vi "SPVM Reader.vi"(8 "error in":errorcluster, 11 "file (use dialog)":path) -> (0 "error out":errorcluster, 1 "VoxelData":u8[](array[numeric]), 3 "Metadata":T1, 4 "Length ( Bytes )":i32, 6 "cancelled":bool)   [LabVIEW 2020]
uses:
  <vilib>/Utility/error.llb/Error Cluster From Error Code.vi
  <vilib>/ErrorRing/Error Ring.xnode
panel:
  out "Scale\nunits":string
  out "Scale\nnumeric":ext
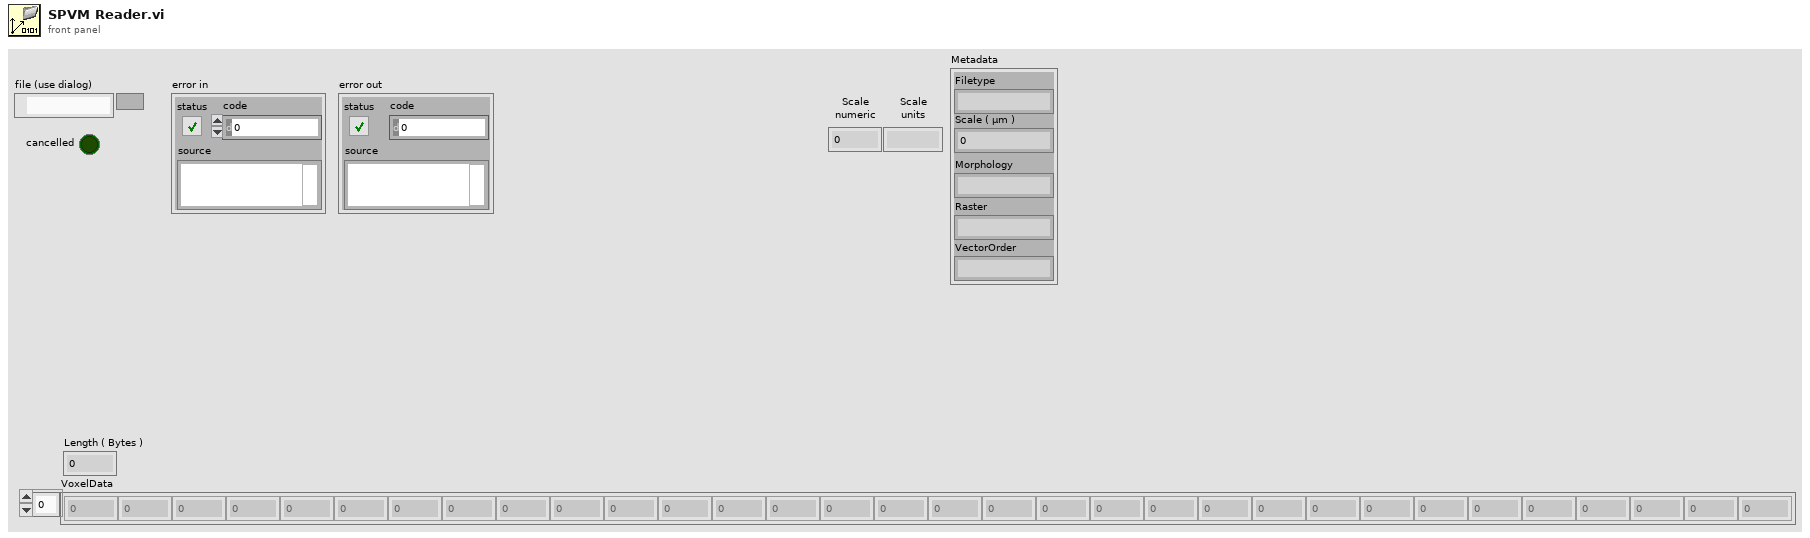
[diagram p1: front panel]
types:
  T1 = cluster{"Filetype":string, "Scale ( µm )":ext, "Morphology":string, "Raster":string, "VectorOrder":string}
  T2 = cluster{"FileType":string, "Scale ( um )":ext, "Morphology":string, "Raster":string, "VectorOrder":string}
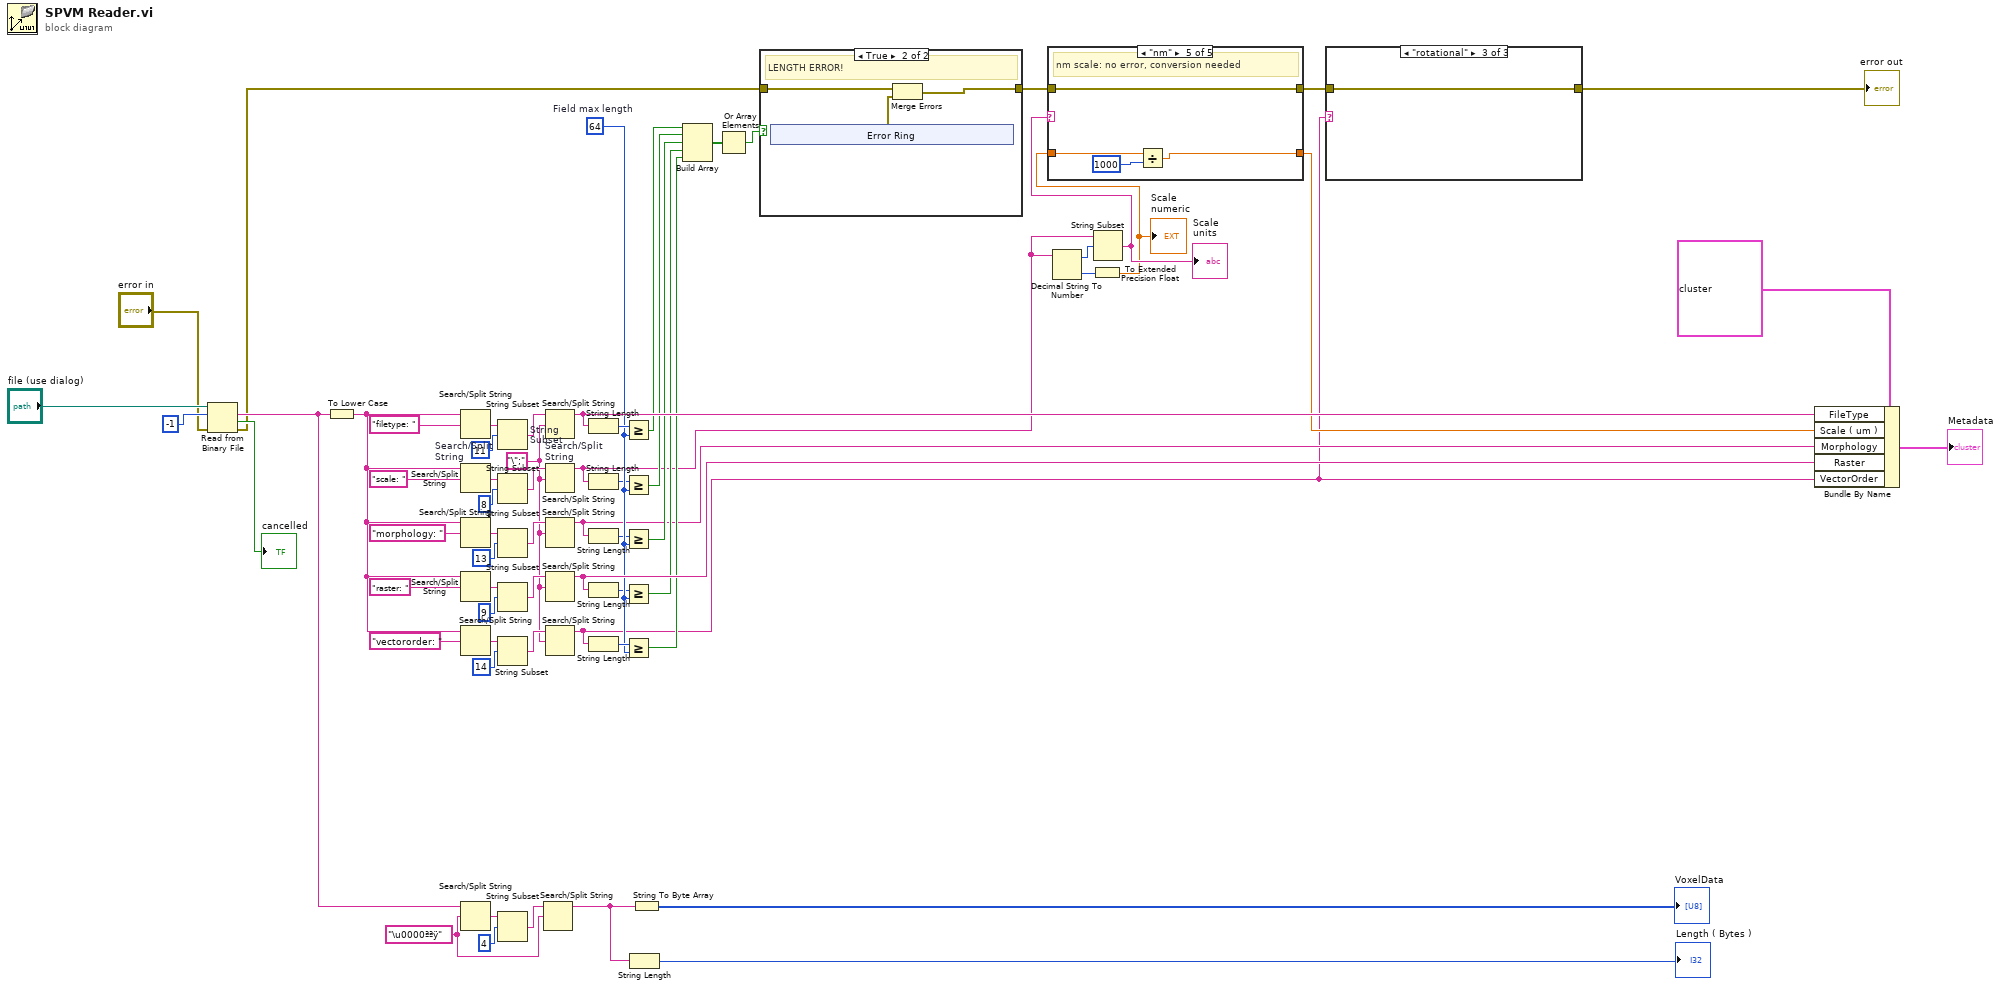
[diagram p0: block diagram]
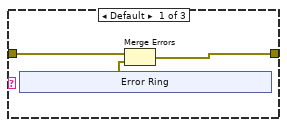
[diagram p2: hidden frame]
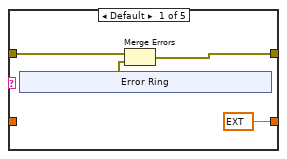
[diagram p4: hidden frame]
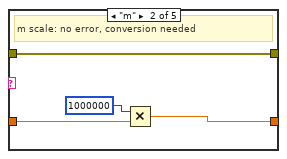
[diagram p5: hidden frame]
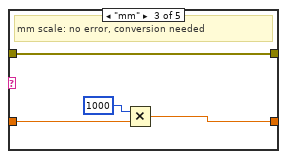
[diagram p6: hidden frame]
diagram:
  w23 = 64  # Field max length
  w29 = "\";" ("search string/char (-)")
  w63 = "\u0000ªªÿ" ("search string/char (-)")
  n1 = Read from Binary File(8:"error in", 10:-1 ("count (1)"), 11:"file (use dialog)") -> (0:w13:errorcluster, 1:→"cancelled":bool, 2:w51:string)  [unwired: 3 in, 1 out]
  n2 = To Lower Case(string=w51) -> (all lower case string=w28:string)
  n3 = Search/Split String "Search/Split\nString"(string=w28, search string/char (-)="filetype: ") -> (match + rest of string=w49:string)  [unwired: 1 in, 2 out]
  n4 = Search/Split String(string=w28, search string/char (-)="scale: ") -> (match + rest of string=w48:string)  [unwired: 1 in, 2 out]
  n5 = Search/Split String(string=w28, search string/char (-)="morphology: ") -> (match + rest of string=w47:string)  [unwired: 1 in, 2 out]
  n6 = Search/Split String(string=w28, search string/char (-)="raster: ") -> (match + rest of string=w46:string)  [unwired: 1 in, 2 out]
  n7 = Search/Split String(string=w28, search string/char (-)="vectororder: ") -> (match + rest of string=w32:string)  [unwired: 1 in, 2 out]
  n8 = Search/Split String(string=w51, search string/char (-)=w63) -> (match + rest of string=w58:string)  [unwired: 1 in, 2 out]
  n9 = String Subset "String\nSubset"(string=w49, offset (0)=11) -> (substring=w38:string)  [unwired: 1 in]
  n10 = String Subset(string=w48, offset (0)=8) -> (substring=w39:string)  [unwired: 1 in]
  n11 = String Subset(string=w47, offset (0)=13) -> (substring=w40:string)  [unwired: 1 in]
  n12 = String Subset(string=w46, offset (0)=9) -> (substring=w41:string)  [unwired: 1 in]
  n13 = String Subset(string=w32, offset (0)=14) -> (substring=w30:string)  [unwired: 1 in]
  n14 = String Subset(string=w58, offset (0)=4) -> (substring=w62:string)  [unwired: 1 in]
  n15 = Search/Split String(string=w62, search string/char (-)=w63) -> (substring before match=w35:string)  [unwired: 1 in, 2 out]
  n16 = Search/Split String "Search/Split\nString"(string=w38, search string/char (-)=w29) -> (substring before match=w27:string)  [unwired: 1 in, 2 out]
  n17 = Search/Split String(string=w39, search string/char (-)=w29) -> (substring before match=w8:string)  [unwired: 1 in, 2 out]
  n18 = Search/Split String(string=w40, search string/char (-)=w29) -> (substring before match=w2:string)  [unwired: 1 in, 2 out]
  n19 = Search/Split String(string=w41, search string/char (-)=w29) -> (substring before match=w26:string)  [unwired: 1 in, 2 out]
  n20 = Search/Split String(string=w30, search string/char (-)=w29) -> (substring before match=w1:string)  [unwired: 1 in, 2 out]
  n21 = String Length(string=w27) -> (length=w25:i32)
  n22 = String Length(string=w8) -> (length=w22:i32)
  n23 = String Length(string=w2) -> (length=w21:i32)
  n24 = String Length(string=w26) -> (length=w20:i32)
  n25 = String Length(string=w1) -> (length=w24:i32)
  n26 = Greater Or Equal?(x=w25, y=w23) -> (x >= y?=w19:bool)
  n27 = Greater Or Equal?(x=w22, y=w23) -> (x >= y?=w18:bool)
  n28 = Greater Or Equal?(x=w21, y=w23) -> (x >= y?=w17:bool)
  n29 = Greater Or Equal?(x=w20, y=w23) -> (x >= y?=w16:bool)
  n30 = Greater Or Equal?(x=w24, y=w23) -> (x >= y?=w15:bool)
  n31 = String Length(string=w35) -> (length=→"Length ( Bytes )":i32)
  n32 = String To Byte Array(string=w35) -> (unsigned byte array=→"VoxelData":u8[])
  n33 = Build Array(w19, w18, w17, w16, w15) -> (w14:bool[])
  n34 = Or Array Elements(Boolean array=w14) -> (logical OR=w12:bool)
  n35 = case shown="True" w12 {
    tunnel: w13 -> [w64 w66]
    tunnel: [w64 w67] -> w10
    frame False {
      # "No length error"
    }
    frame True {
      # "LENGTH ERROR!"
      n36 = xnode "Error Ring"() -> ("error out"=w65:errorcluster)
      n37 = Merge Errors(w66, w65) -> (w67:errorcluster)
    }
  }
  n38 = Decimal String To Number(string=w8) -> (offset past number=w11:i32, number=w9:i32)  [unwired: 2 in]
  n39 = String Subset(string=w8, offset (0)=w11) -> (substring=w6:string)  [unwired: 1 in]
  "Scale\nunits" <- w6
  n40 = To Extended Precision Float(1:w9) -> (0:w5:ext)
  "Scale\nnumeric" <- w5
  n41 = case shown="\"nm\"" w6 {
    tunnel: [ext nan w85 w89 w91 w92] -> w7
    tunnel: w5 -> [_ w84 w88 w91 w94]
    tunnel: w10 -> [w75 w82 w86 w90 w95]
    tunnel: [w76 w82 w86 w90 w95] -> w4
    frame Default {
      n42 = xnode "Error Ring"() -> ("error out"=w74:errorcluster)
      n43 = Merge Errors(w75, w74) -> (w76:errorcluster)
    }
    frame "m" {
      # "m scale: no error, conversion needed"
      n44 = Multiply(x=1000000, y=w84) -> (x*y=w85:ext)
    }
    frame "mm" {
      # "mm scale: no error, conversion needed"
      n45 = Multiply(x=1000, y=w88) -> (x*y=w89:ext)
    }
    frame "µm" {
      # "µm scale: no error, no conversion needed"
    }
    frame "nm" {
      # "nm scale: no error, conversion needed"
      n46 = Divide(x=w94, y=1000 ("x")) -> (x/y=w92:ext)
    }
  }
  n47 = case shown="\"rotational\"" w1 {
    tunnel: w4 -> [w97 w104 w105]
    tunnel: [w98 w104 w105] -> w3
    frame Default {
      n48 = xnode "Error Ring"() -> ("error out"=w96:errorcluster)
      n49 = Merge Errors(w97, w96) -> (w98:errorcluster)
    }
    frame "planar" {
    }
    frame "rotational" {
    }
  }
  "error out" <- w3
  n50 = Bundle By Name "Bundle By Name"(cluster=T2 {"FileType"="", "Scale ( um )"=0.0, "Morphology"="", "Raster"="", "VectorOrder"=""} ("input cluster"), "FileType"=w27, "Scale ( um )"=w7, "Morphology"=w2, "Raster"=w26, "VectorOrder"=w1) -> (→"Metadata":T2)
